vi "Send Online Update.vi"(8 "error in (no error)":errorcluster, 11 "Server in":refnum<class "Server.lvclass">) -> (0 "error out":errorcluster, 3 "Server out":refnum<class "Server.lvclass">)   [LabVIEW 2018]
uses:
  Chat Window Model/Chat Window Model Messages/Update Online List Msg/Update Online List Msg.lvclass
  Chat Window Register (Class)/Chat Window Register.lvclass
  Server.lvclass
  C:/Program Files (x86)/National Instruments/LabVIEW 2018/vi.lib/ActorFramework/Actor/Actor.lvclass
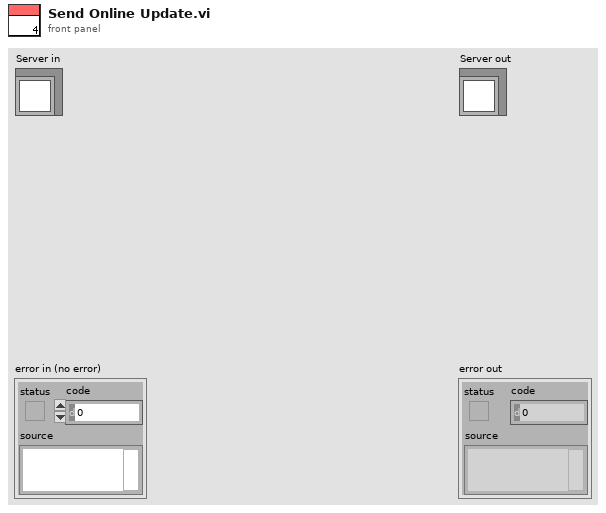
[diagram p1: front panel]
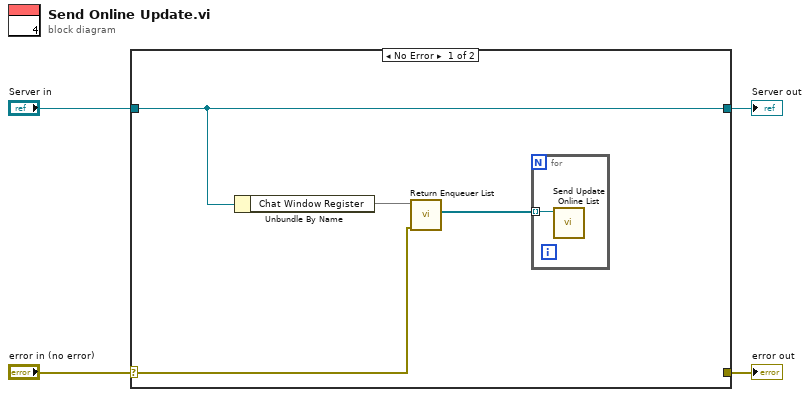
[diagram p0: block diagram]
diagram:
  n1 = case shown="No Error" "error in (no error)" {
    selector: "error in (no error)" -> [w6 w11]
    tunnel: [_ w11] -> w3
    tunnel: [w8 w10] -> w1
    tunnel: "Server in" -> [w8 w10]
    frame No Error {
      n2 = Unbundle By Name(w8) -> ("Chat Window Register"=w7)
      n3 = call "Return Enqueuer List.vi"("error in (no error)"=w6, "Chat Window Register in"=w7) -> ("Chat Window Enqueuers"=w5:refnum<class "Message Enqueuer.lvclass">[])  [unwired: 7 in, 2 out]
      n4 = for {
        tunnel: w5 -> [w9] mode=indexing
        n5 = call "Send Update Online List.vi"("Message Enqueuer"=w9) -> ()  [unwired: 9 in, 2 out]
      }
    }
    frame Error {
    }
  }
  "error out" <- w3
  "Server out" <- w1
